vi "CreateNewFile.vi"(9 "File Name":string, 10 ".note path":path, 11 "Folder":path) -> (1 "Current file":string, 2 ".note file refnum":refnum<file>, 3 "Byte Stream File refnum":refnum<file>)   [LabVIEW 2011]
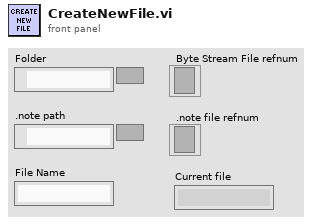
[diagram p1: front panel]
types:
  T1 = enum16{"open", "replace", "create", "open or create", "replace or create", "replace or create with confirmation"}
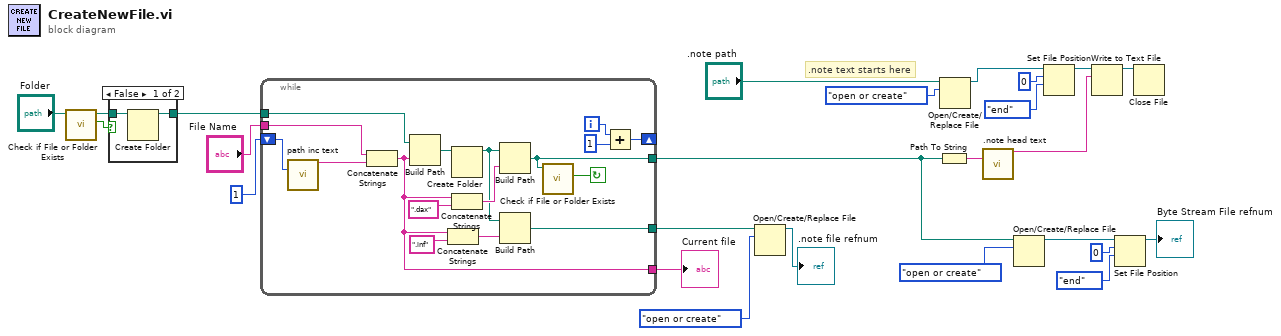
[diagram p0: block diagram]
diagram:
  # ".note text starts here"
  n1 = call <vilib>:"Check if File or Folder Exists.vi"("path"="Folder") -> ("file or folder exists?"=w17:bool, "dup path"=w16:path)  [unwired: 8 in, 1 out]
  n2 = case shown="False" w17 {
    tunnel: [w27 w28] -> w18
    tunnel: w16 -> [w26 w28]
    frame False {
      n3 = Create Folder(path (use dialog)=w26) -> (created path=w27:path)  [unwired: 2 in, 2 out]
    }
    frame True {
    }
  }
  n4 = while {
    tunnel: [w44] -> w23
    shift-right: [w39] -> _
    shift-left: 1 -> [w45]
    tunnel: w18 -> [w33]
    tunnel: [w34] -> w21
    tunnel: "File Name" -> [w30]
    tunnel: [w29] -> w22
    i -> [w41]
    stop <- w43 continue-if-true
    n5 = call "path inc text"("inc"=w45) -> ("Result"=w42:string)  [unwired: 13 in, 1 out]
    n6 = Concatenate Strings(w30, w42) -> (w29:string)
    n7 = Build Path(base path=w33, name or relative path=w29) -> (appended path=w32:path)
    n8 = Concatenate Strings(w29, ".inf" ("string")) -> (w35:string)
    n9 = Create Folder(path (use dialog)=w32) -> (created path=w31:path)  [unwired: 2 in, 2 out]
    n10 = Concatenate Strings(w29, ".dax" ("string")) -> (w37:string)
    n11 = Build Path(base path=w31, name or relative path=w37) -> (appended path=w44:path)
    n12 = Build Path(base path=w31, name or relative path=w35) -> (appended path=w34:path)
    n13 = call <vilib>:"Check if File or Folder Exists.vi"("path"=w44) -> ("file or folder exists?"=w43:bool)  [unwired: 8 in, 2 out]
    n14 = Add(x=w41, y=1) -> (x+y=w39:i32)
  }
  "Current file" <- w22
  n15 = Open/Create/Replace File(file path (use dialog)=w21, operation (0:open)=T1."open or create") -> (refnum out=→".note file refnum":refnum<file>)  [unwired: 4 in, 2 out]
  n16 = Path To String(path=w23) -> (string=w1:string)
  n17 = Open/Create/Replace File(file path (use dialog)=".note path", operation (0:open)=T1."open or create") -> (refnum out=w5:refnum<file>)  [unwired: 4 in, 2 out]
  n18 = call ".note head text"(".daxfilepath"=w1) -> ("Result"=w2:string)  [unwired: 13 in, 1 out]
  n19 = Open/Create/Replace File(file path (use dialog)=w23, operation (0:open)=T1."open or create") -> (refnum out=w13:refnum<file>)  [unwired: 4 in, 2 out]
  n20 = Set File Position(offset (in bytes) (0)=i64 0, refnum=w5, from (0:start)=enum16{"start", "end", "current"}."end") -> (refnum out=w4:refnum<file>)  [unwired: 1 in, 1 out]
  n21 = Write to Text File(file (use dialog)=w4, text=w2) -> (refnum out=w3:refnum<file>)  [unwired: 2 in, 2 out]
  n22 = Set File Position(offset (in bytes) (0)=i64 0, refnum=w13, from (0:start)=enum16{"start", "end", "current"}."end") -> (refnum out=→"Byte Stream File refnum":refnum<file>)  [unwired: 1 in, 1 out]
  n23 = Close File(refnum=w3) -> ()  [unwired: 1 in, 2 out]
